vi "HatchLatchToDash.vi"(10 "Update?":bool, 11 "HatchLatchIn":bool) -> (3 "HatchLatchOut":bool)   [LabVIEW 2018]
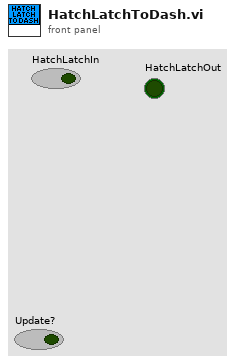
[diagram p1: front panel]
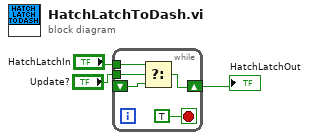
[diagram p0: block diagram]
diagram:
  n1 = while {
    tunnel: "Update?" -> [w8]
    shift-right: [w7] -> w1
    shift-left: _ -> [w6]
    tunnel: "HatchLatchIn" -> [w4]
    stop <- TRUE stop-if-true
    n2 = Select(t=w4, s=w8, f=w6) -> (s? t:f=w7:bool)
  }
  "HatchLatchOut" <- w1
